vi "NOSAMSNoBouncerDAQrestartFC.vi"(8 "error in (no error)":errorcluster) -> (0 "error out":errorcluster, 2 "Summary Data":T3={"C12LE"=1.472651644671806e-07, "C13LE"=7.43208703350402e-08, "C12"=7.325707563373238e-08, "C13L"=240.0, "C13H"=6.302996266666667, "C1312"=6.305409493333333, "Counts"=0, "LT"=1.0021241544060013, "RT"=0.0, "BadBlocks"=0}, 3 "Run Average Ratios":T7={"C14Rate"=38.07712869341802, "CountErr"=0.06454972243679029, "DT"=0.002413226666666546, "DTfrac"=0.0003827232266545153, "C13"=307109705561.01575, "C13H/L"=0.9856864606602128, "d13C"=-48.24793286826845, "C14/13"=1.23985429323571e-10, "C12Cor"=28715190239906.207, "C13/12"=0.010695028328772694, "C14/12"=1.3260273874313845e-12, "LEC13/12"=0.0} {"LEC13/12" format="%_4e"; "DTfrac" format="%#_3g"; "DT" format="%#_3g"; "CountErr" format="%#_3g"; "d13C" format="%_4g"; "C13/12" format="%_4e"; "C14/12" format="%_4e"; "C14/13" format="%_3e"; "C12Cor" format="%_3e"; "C13" format="%_3e"; "C13H/L" format="%#_3g"})   [LabVIEW 2013]
uses:
  PixieKeithleyDAQstates.ctl
  <vilib>/DAQmx/configure/timing.llb/DAQmx Timing (Sample Clock).vi
  <vilib>/DAQmx/create/channels.llb/DAQmx Create Channel (AI-Voltage-Basic).vi
  <vilib>/DAQmx/create/channels.llb/DAQmx Create Channel (CI-Count Edges).vi
  <vilib>/DAQmx/read.llb/DAQmx Read (Counter U32 1Chan 1Samp).vi
  <resource>/objmgr/daqmx.rc
  <vilib>/DAQmx/configure/trigger.llb/DAQmx Start Trigger (Digital Edge).vi
  <vilib>/DAQmx/read.llb/DAQmx Read (Analog 1D Wfm NChan NSamp).vi
  <vilib>/DAQmx/write.llb/DAQmx Write (Analog Wfm 1Chan NSamp).vi
  <vilib>/DAQmx/create/channels.llb/DAQmx Create Channel (AO-Voltage-Basic).vi
  <vilib>/DAQmx/configure/timing.llb/DAQmx Timing (Use Waveform).vi
  <vilib>/DAQmx/configure/timing.llb/DAQmx Timing (Implicit).vi
  <vilib>/DAQmx/create/channels.llb/DAQmx Create Channel (CO-Pulse Generation-Time).vi
  RunRatios.ctl
  FCOffset.ctl
  SummaryData.ctl
  BouncerParameters.ctl
panel:
  out "Waveform Chart":waveform(dbl)[](graph)
  out "Bouncer Waveform":waveform(dbl)(graph)
  in  "Bouncer Parameters":T1={"12C Period"=1.0, "12C Delay"=0.0, "12C Voltage"=9.022, "13C Period"=10.0, "13C Delay"=0.0, "13C Voltage"=5.239, "14C Period"=100.0, "14C Delay"=0.0, "14C Voltage"=2.0, "LE13C Period"=0.0, "LE13C Delay"=0.0, "LE13C Voltage"=0.0, "LE12C Period"=0.0, "LE12C Delay"=0.0, "LE12C Voltage"=0.0} {"LE12C Voltage" format="%_4f"; "LE13C Voltage" format="%_4f"}
  out "CH1 GDT":dbl
  out "CH0 GDT":dbl
  in  "FC Offset":T2={"HE 12C Offset"=0.0, "HE 13CL Offset"=0.0, "HE 13CH Offset"=0.0, "LE FC Scale"=0, "HE C12 Scale"=0, "HE C13 Scale"=18} {"HE C13 Scale" items=["500 mA/V", "200 mA/V", "100 mA/V", "50 mA/V", "20 mA/V", "10 mA/V", "5 mA/V", "2 mA/V", "1 mA/V", "500 uA/V", "200 uA/V", "100 uA/V", "50 uA/V", "20 uA/V", "10 uA/V", "5 uA/V", "2 uA/V", "1 uA/V", "500 nA/V", "200 nA/V", "100 nA/V", "50 nA/V", "20 nA/V", "10 nA/V", "5 nA/V", "2 nA/V", "1 nA/V", "500 pA/V", "200 pA/V", "100 pA/V", "50 pA/V", "20 pA/V", "10 pA/V", "5 pA/V", "2 pA/V", "1 pA/V", ""]; "HE C12 Scale" items=["500 mA/V", "200 mA/V", "100 mA/V", "50 mA/V", "20 mA/V", "10 mA/V", "5 mA/V", "2 mA/V", "1 mA/V", "500 uA/V", "200 uA/V", "100 uA/V", "50 uA/V", "20 uA/V", "10 uA/V", "5 uA/V", "2 uA/V", "1 uA/V", "500 nA/V", "200 nA/V", "100 nA/V", "50 nA/V", "20 nA/V", "10 nA/V", "5 nA/V", "2 nA/V", "1 nA/V", "500 pA/V", "200 pA/V", "100 pA/V", "50 pA/V", "20 pA/V", "10 pA/V", "5 pA/V", "2 pA/V", "1 pA/V", ""]; "LE FC Scale" items=["500 mA/V", "200 mA/V", "100 mA/V", "50 mA/V", "20 mA/V", "10 mA/V", "5 mA/V", "2 mA/V", "1 mA/V", "500 uA/V", "200 uA/V", "100 uA/V", "50 uA/V", "20 uA/V", "10 uA/V", "5 uA/V", "2 uA/V", "1 uA/V", "500 nA/V", "200 nA/V", "100 nA/V", "50 nA/V", "20 nA/V", "10 nA/V", "5 nA/V", "2 nA/V", "1 nA/V", "500 pA/V", "200 pA/V", "100 pA/V", "50 pA/V", "20 pA/V", "10 pA/V", "5 pA/V", "2 pA/V", "1 pA/V", ""]}
  out "HE 13CL Cup":waveform(dbl)(graph)={"t0"=timestamp(3415120333.4017754 s since 1904-01-01), "dt"=9.999999999999972e-06, "Y"=[0.41889009921070675, 0.6410939957678486, 0.7270772818431984, 0.7261111773784867, 0.7270772818431984, 0.7293315256055366, 0.7267552470213039, 0.7286874559575331, 0.7306196649054364, 0.7254671077369653, 0.7283654211340178, 0.7302976300799747, 0.7277213514879598, 0.7261111773784867, 0.7306196649054364, 0.7341620480069433, 0.7293315256055366, 0.7302976300799747, 0.7319078042105287, 0.7331959435208164, 0.7280433863108267, 0.7331959435208164, 0.7290094907813727, 0.7299755952548376, 0.7309416997312226, 0.7344840828363023, 0.7293315256055366, 0.7299755952548376, 0.7267552470213039, 0.7338400131779094, 0.7219247247317432, 0.7225687943661443, 0.7280433863108267, 0.7280433863108267, 0.7309416997312226, 0.7290094907813727, 0.7328739086927573, 0.7277213514879598, 0.7161280980802982, 0.7286874559575331], "attributes"=variant("NI_ChannelName"=variant(string "PXI1Slot2/ai2"), "NI_UnitDescription"=variant(string "Volts"))}
  out "Bouncer":waveform(dbl)(graph)={"t0"=timestamp(3415120333.4009705 s since 1904-01-01), "dt"=9.999999999999972e-06, "Y"=array[1000 elements], "attributes"=variant("NI_ChannelName"=variant(string "PXI1Slot2/ai0"), "NI_UnitDescription"=variant(string "Volts"))}
  out "LE 13C Cup":waveform(dbl)(graph)={"t0"=timestamp(3415120333.402178 s since 1904-01-01), "dt"=9.999999999999972e-06, "Y"=[0.8050097183722652, 0.24660166407635983, 0.028584441505206795, 0.009584422869030943, 0.009906457076575987, 0.00797425183471986, 0.00797425183471986, 0.007008149216862962, 0.012804764954733521, 0.01312679916455761, 0.010550525492349248, 0.010872559700577551, 0.009584422869030943, 0.01022849128434874, 0.01151662811771772, 0.010872559700577551, 0.010872559700577551, 0.010872559700577551, 0.01022849128434874, 0.009262388661713566, 0.004109841375562904, 0.009262388661713566, 0.01151662811771772, 0.01022849128434874, 0.019567483409006912, 0.01151662811771772, 0.010872559700577551, 0.009906457076575987, 0.009584422869030943, 0.01022849128434874, 0.013448833374609843, 0.01022849128434874, 0.009906457076575987, 0.010550525492349248, 0.00668611501136536, 0.010550525492349248, 0.01022849128434874, 0.01022849128434874, 0.009584422869030943, 0.013448833374609843], "attributes"=variant("NI_ChannelName"=variant(string "PXI1Slot2/ai3"), "NI_UnitDescription"=variant(string "Volts"))}
  out "LE 12C Cup":waveform(dbl)(graph)={"t0"=timestamp(3415120333.4013777 s since 1904-01-01), "dt"=9.999999999999972e-06, "Y"=[0.00668611501136536, 0.007008149216862962, 0.007652217628540168, 0.007330183422587883, 0.00861832024776164, 0.007330183422587883, 0.009262388661713566, 0.01312679916455761, 0.05338107720327494, 0.6781279926088322, 0.8175690797952145, 0.8223996035554544, 0.8240097781590372, 0.8233657083165931, 0.8249758829252316, 0.8230436733958766, 0.8243318130807649, 0.8236877432376466, 0.8243318130807649, 0.8243318130807649, 0.8233657083165931, 0.8278741972420289, 0.8236877432376466, 0.8240097781590372, 0.8227216384754971, 0.8246538480028296, 0.8246538480028296, 0.8246538480028296, 0.8249758829252316, 0.8252979178479707, 0.8214334987973474, 0.8236877432376466, 0.8246538480028296, 0.8246538480028296, 0.8227216384754971, 0.8236877432376466, 0.8243318130807649, 0.8217555337163797, 0.8240097781590372, 0.8243318130807649], "attributes"=variant("NI_ChannelName"=variant(string "PXI1Slot2/ai3"), "NI_UnitDescription"=variant(string "Volts"))}
  out "HE 13CH Cup":waveform(dbl)(graph)={"t0"=timestamp(3415120333.4017754 s since 1904-01-01), "dt"=9.999999999999972e-06, "Y"=[0.41889009921070675, 0.6410939957678486, 0.7270772818431984, 0.7261111773784867, 0.7270772818431984, 0.7293315256055366, 0.7267552470213039, 0.7286874559575331, 0.7306196649054364, 0.7254671077369653, 0.7283654211340178, 0.7302976300799747, 0.7277213514879598, 0.7261111773784867, 0.7306196649054364, 0.7341620480069433, 0.7293315256055366, 0.7302976300799747, 0.7319078042105287, 0.7331959435208164, 0.7280433863108267, 0.7331959435208164, 0.7290094907813727, 0.7299755952548376, 0.7309416997312226, 0.7344840828363023, 0.7293315256055366, 0.7299755952548376, 0.7267552470213039, 0.7338400131779094, 0.7219247247317432, 0.7225687943661443, 0.7280433863108267, 0.7280433863108267, 0.7309416997312226, 0.7290094907813727, 0.7328739086927573, 0.7277213514879598, 0.7161280980802982, 0.7286874559575331], "attributes"=variant("NI_ChannelName"=variant(string "PXI1Slot2/ai2"), "NI_UnitDescription"=variant(string "Volts"))}
  out "HE 12C Cup":waveform(dbl)(graph)={"t0"=timestamp(3415120333.400973 s since 1904-01-01), "dt"=9.999999999999972e-06, "Y"=[-0.00168677425192447, 0.003143738765882537, -0.002652876849375083, -0.00168677425192447, 0.0008894993512310448, -0.002652876849375083, 0.0005674651500443148, -0.000720671652438485, 0.0018556019561503992, 0.0018556019561503992, 0.0024996703605630385, 0.0015335677542840436, 0.002177636158243383, -0.0013647400523220184, 0.005397978191647298, 0.0018556019561503992, 0.0012115335526442733, 0.0015335677542840436, 0.016669175487689536, 0.2607711773435167, 0.6375516136789285, 0.6369075442122739, 0.6423821347186465, 0.6456024821175347, 0.6449584126352536, 0.6423821347186465, 0.6456024821175347, 0.6427041694571275, 0.639805856822051, 0.6427041694571275, 0.6388397526159826, 0.6449584126352536, 0.6423821347186465, 0.6443143431542244, 0.6452804473762376, 0.6401278915580318, 0.6410939957678486, 0.6468906210858548, 0.6446363778945825, 0.6433482389350278], "attributes"=variant("NI_ChannelName"=variant(string "PXI1Slot2/ai1"), "NI_UnitDescription"=variant(string "Volts"))}
  out "C13LE":dbl=7.360825676338929e-08 format="%_4g"
  out "C12LE":dbl=7.360825676338929e-08 format="%_4g"
  in  "SampClk.Rate":dbl=10000.0
  out "DT Corrected Rate":dbl=38.103932081925684
  out "SCA Rate":dbl=38.473667612740456
  out "SCA Counts":u32=244
  out "CH1 SFDT":dbl=0.004433706666666666 format="%#_2f"
  out "CH0 SFDT":dbl=0.004324053333333333 format="%#_2f"
  in  "Mode":enum16{"Tuning", "Run", "Manual"}(ring)
  out "Block Spectrum":u32[][](graph) caption="ADC Spectrum"
  out "RunningAverages":T3={"C12LE"=1.4726514132603862e-07, "C13LE"=7.431122697335651e-08, "C12"=7.326197420828519e-08, "C13L"=222.0, "C13H"=5.887767893333334, "C1312"=5.884231466666667, "Counts"=0, "LT"=1.0020921000294485, "RT"=0.0, "BadBlocks"=0}
  out "Elapsed Time":dbl=6.3420000000000005
  out "element":T4=enum."Idle"
  in  "Stop":bool
  in  "Stop DAQ":bool
  in  "Run Parameters":T5={"Block time (s)"=0.2, "Max Runtime (s)"=100000.0, "Max Counts"=100000, "C12 Limit"=-1.0, "Max BadBlocks"=100} {"Block time (s)" min=0.0 max=100.0 step=0.1}
  out "Acquiring":bool
  in  "StartDAQ":bool
  in  "Logfile":string="Feb12.txt"
  in  "Log File Path":path=path "C:/DAQ Logs"
  out "Good Block":bool=TRUE
  out "Currents & Counts":cluster{dbl, dbl, dbl, dbl, dbl}(graph)
  out "Ratios":T6(graph)={"C14/12"=1.3260273874313845e-12, "C14/12"=1.3130784198635677e-12, "d13C"=-48.24793286826845, "d13C"=-48.27837602145524}
  out "13C H/L":dbl(knob)=0.9886607752123965 scale=0.0..2.0 scale format="%#_3g"
  out "Currents":cluster{dbl, dbl}(knob)={1.4754487124301994e-07, 1.4806074705013686e-07} scale=0.0..1e-06 scale format="%#_1e"
  out "12/13":dbl=93.50437948492602
  out "Ch1 Rate 2":cluster{dbl, "Ch1 Rate":dbl}(graph)={38.07712869341802, "Ch1 Rate"=37.7052907013146}
  out "Moving Averages":T7={"C14Rate"=37.7052907013146, "CountErr"=0.06711560552140243, "DT"=-0.0035364266666668698, "DTfrac"=-0.0006010006041910865, "C13"=307099831658.9964, "C13H/L"=0.9858802928197172, "d13C"=-48.27837602145524, "C14/13"=1.2277861077821284e-10, "C12Cor"=28715185727621.875, "C13/12"=0.010694686232971703, "C14/12"=1.3130784198635677e-12, "LEC13/12"=0.0} {"LEC13/12" format="%_4e"; "DTfrac" format="%#_3g"; "DT" format="%#_3g"; "CountErr" format="%#_3g"; "d13C" format="%_4g"; "C13/12" format="%_4e"; "C14/12" format="%_4e"; "C14/13" format="%_3e"; "C12Cor" format="%_3e"; "C13" format="%_3e"; "C13H/L" format="%#_3g"}
  in  "CountPoints":i32=30 min=1
  in  "CurPoints":i32=30 min=1
  out "C12":dbl=1.4754487124301994e-07 format="%_4g"
  out "C13L":dbl=7.445249028674759e-08 format="%_4g"
  out "C13H":dbl=7.360825676338929e-08 format="%_4g"
  out "Run time [s]":dbl=6.305409493333333 format="%_6g"
  out "Ch1 LT":dbl=6.302996266666667
  out "Ch1 Counts":u32=240
  out "Ch1 Rate":dbl=38.07712869341802
  out "Ch0 LT":dbl=6.305354879999999
  out "Ch0 Counts":u32=243
  out "Ch0 Rate":dbl=38.53867143477895
  # "Currents"
  # "Counts"
  # "Livetime"
  # "Rate"
  # "SFDT"
  # "GDT"
  # "Cor Rate"
  # "Ch 0"
  # "Ch1"
  # "SCA"
  # "ms"
  # "us"
  # "kV"
  # "ms"
  # "us"
  # "kV"
  # "ms"
  # "us"
  # "kV"
  # "ms"
  # "us"
  # "kV"
  # "ms"
  # "us"
  # "kV"
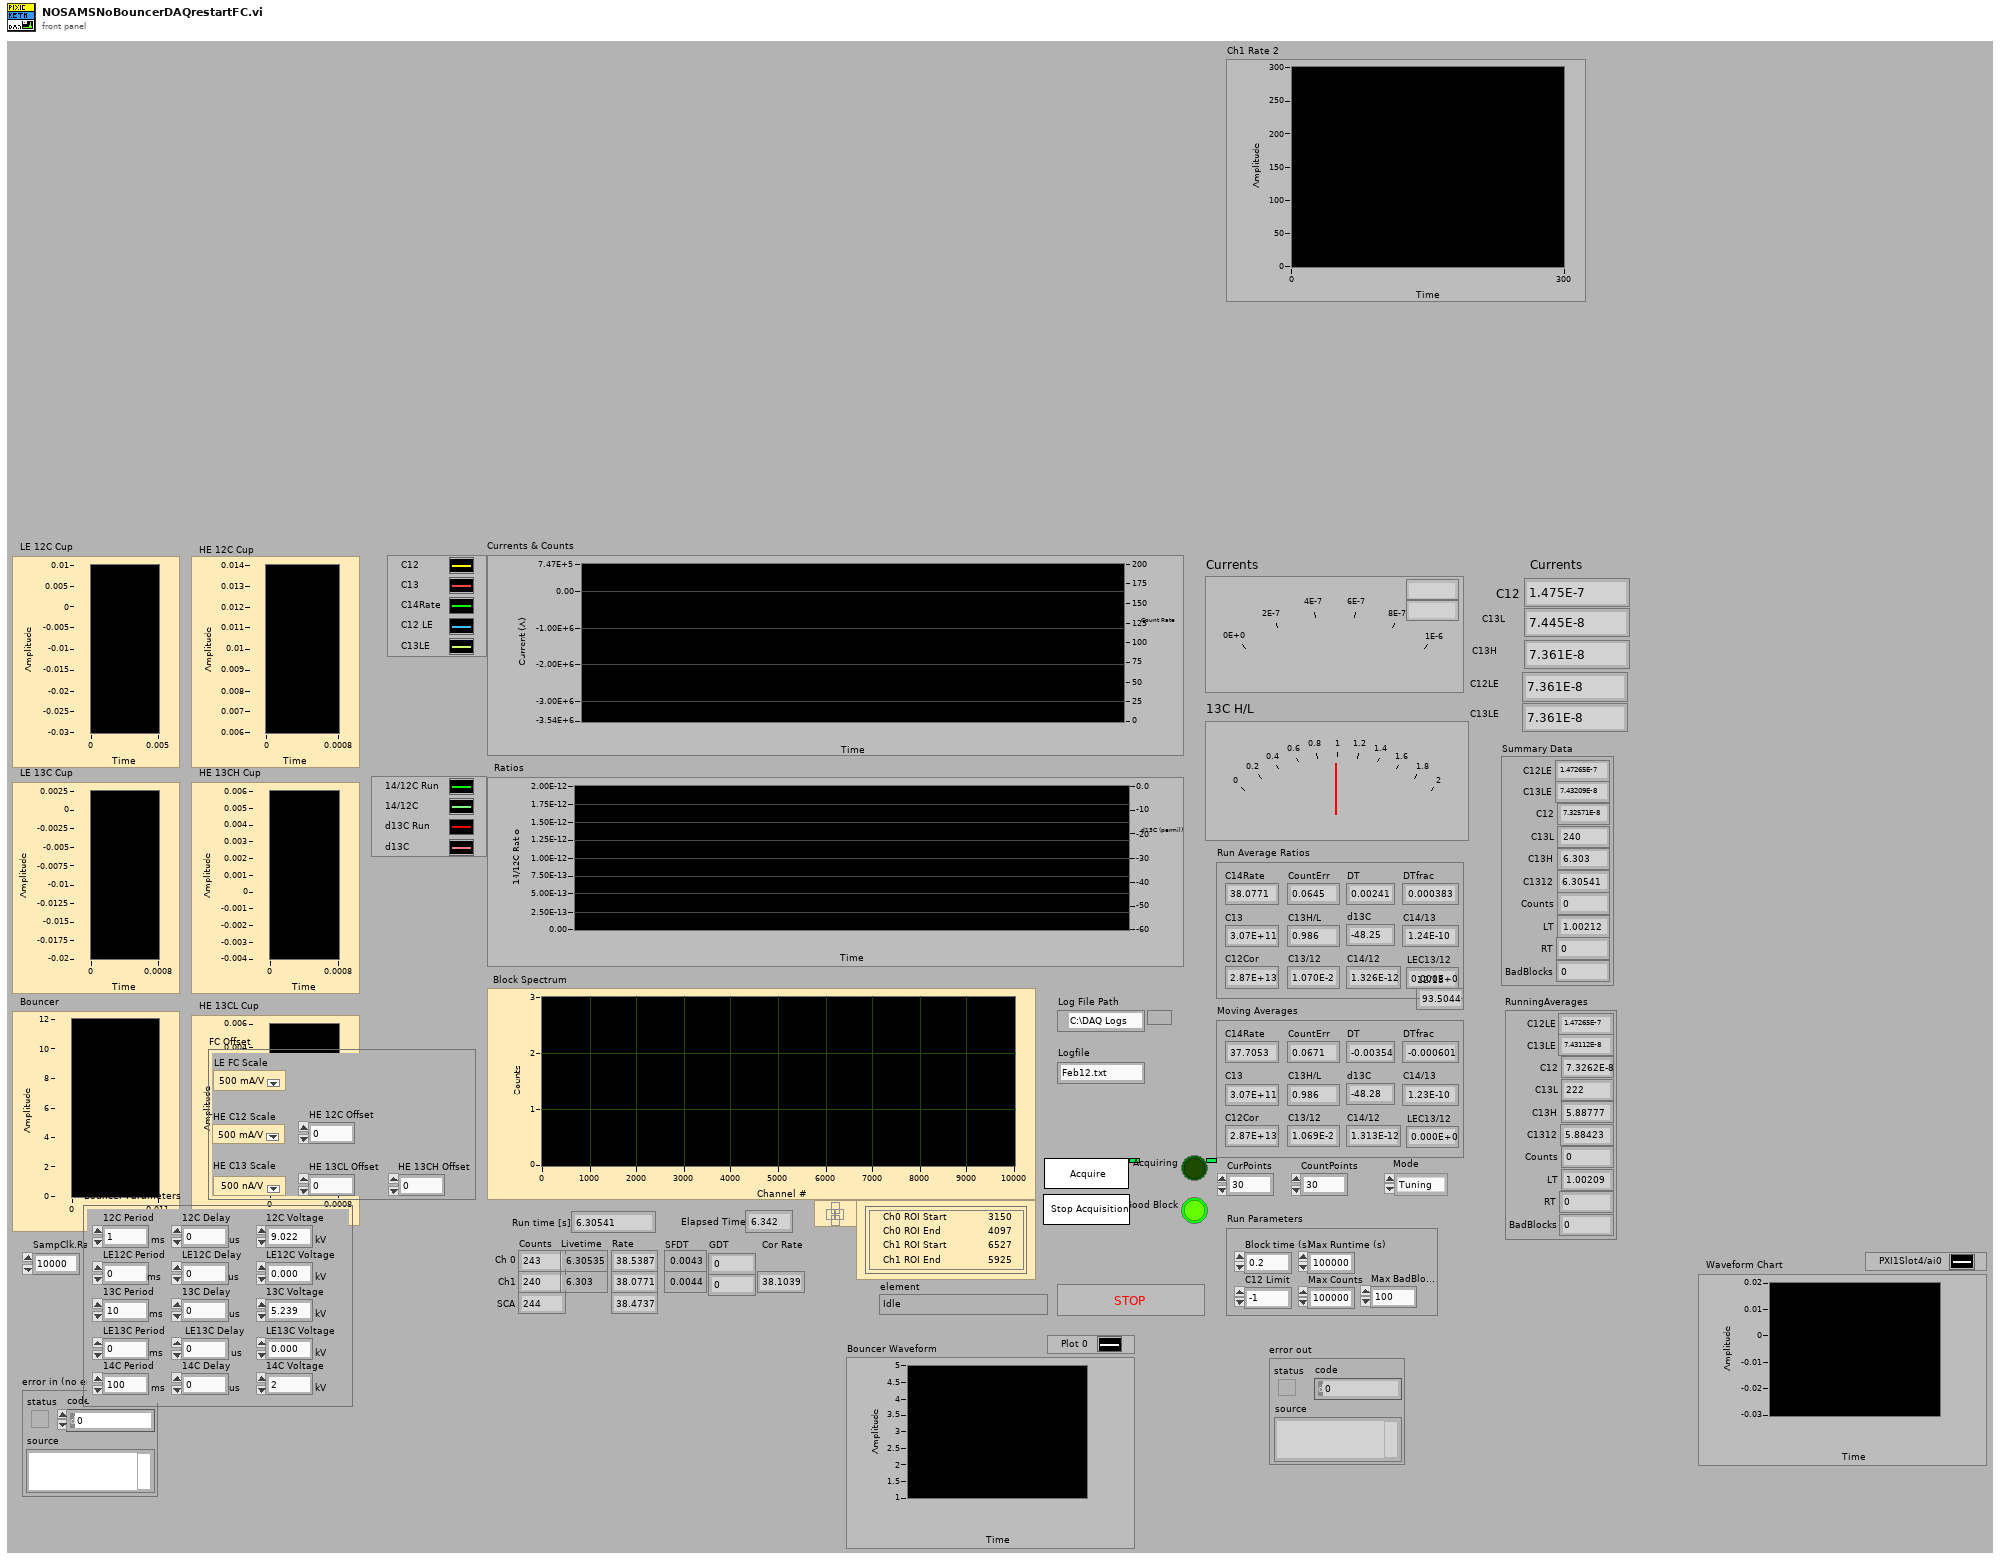
[diagram p1: front panel]
types:
  T1 = typedef "BouncerParameters.ctl" = cluster{"12C Period":dbl, "12C Delay":dbl, "12C Voltage":dbl, "13C Period":dbl, "13C Delay":dbl, "13C Voltage":dbl, "14C Period":dbl, "14C Delay":dbl, "14C Voltage":dbl, "LE13C Period":dbl, "LE13C Delay":dbl, "LE13C Voltage":dbl, "LE12C Period":dbl, "LE12C Delay":dbl, "LE12C Voltage":dbl}
  T2 = typedef "FCOffset.ctl" = cluster{"HE 12C Offset":dbl, "HE 13CL Offset":dbl, "HE 13CH Offset":dbl, "LE FC Scale":u16, "HE C12 Scale":u16, "HE C13 Scale":u16}
  T3 = typedef "SummaryData.ctl" = cluster{"C12LE":dbl, "C13LE":dbl, "C12":dbl, "C13L":dbl, "C13H":dbl, "C1312":dbl, "Counts":u32, "LT":dbl, "RT":dbl, "BadBlocks":u8}
  T4 = typedef "PixieKeithleyDAQstates.ctl" = enum16{"Initialize", "Restart Bouncer", "Idle", "Load Wheel", "Load Sample", "Start Run", "Wait", "Get Block", "Check Data", "Check Run", "Check Sample", "Analyse and Display", "Stop DAQ", "Log Data", "Stop"}
  T5 = cluster{"Block time (s)":dbl, "Max Runtime (s)":dbl, "Max Counts":u32, "C12 Limit":dbl, "Max BadBlocks":u8}
  T6 = cluster{"C14/12":dbl, "C14/12":dbl, "d13C":dbl, "d13C":dbl}
  T7 = typedef "RunRatios.ctl" = cluster{"C14Rate":dbl, "CountErr":dbl, "DT":dbl, "DTfrac":dbl, "C13":dbl, "C13H/L":dbl, "d13C":dbl, "C14/13":dbl, "C12Cor":dbl, "C13/12":dbl, "C14/12":dbl, "LEC13/12":dbl}
  T8 = typedef "BlockData.ctl" = cluster{"LE C12":dbl[], "LE C13":dbl[], "C12":dbl[], "C13L":dbl[], "C13H":dbl[], "C1312":dbl[], "Counts":u32[], "LT":dbl[], "RT":dbl[]}
  T9 = typedef "PixieTimes.ctl" = cluster{"CH0 LT":dbl, "CH1 LT":dbl, "CH0 SFDT":dbl, "CH1 SFDT":dbl, "CH0 GDT":dbl, "CH1 GDT":dbl, "Run time [s]":dbl}
  T10 = typedef "LVCursorListTypeDef.ctl" = cluster{"Name":string, "Color":u32, "Style":u8, "Point Style":u8, "Name Visible":bool, "Allow Drag":bool, "Cursor Mode":u32, "Plot":i32, "Index":i32, "Position":cluster{"X":dbl, "Y":dbl}, "X Scale":u32, "Y Scale":u32, "Watch Plots":i32[], "Watch All Plots":bool, "Plot Area":i32, "Label Offset":cluster{"X":dbl, "Y":dbl}}[]
  T11 = cluster{"Ch0 Counts":u32, "Ch0 Rate":dbl, "Ch1 Counts":u32, "Ch1 Rate":dbl}
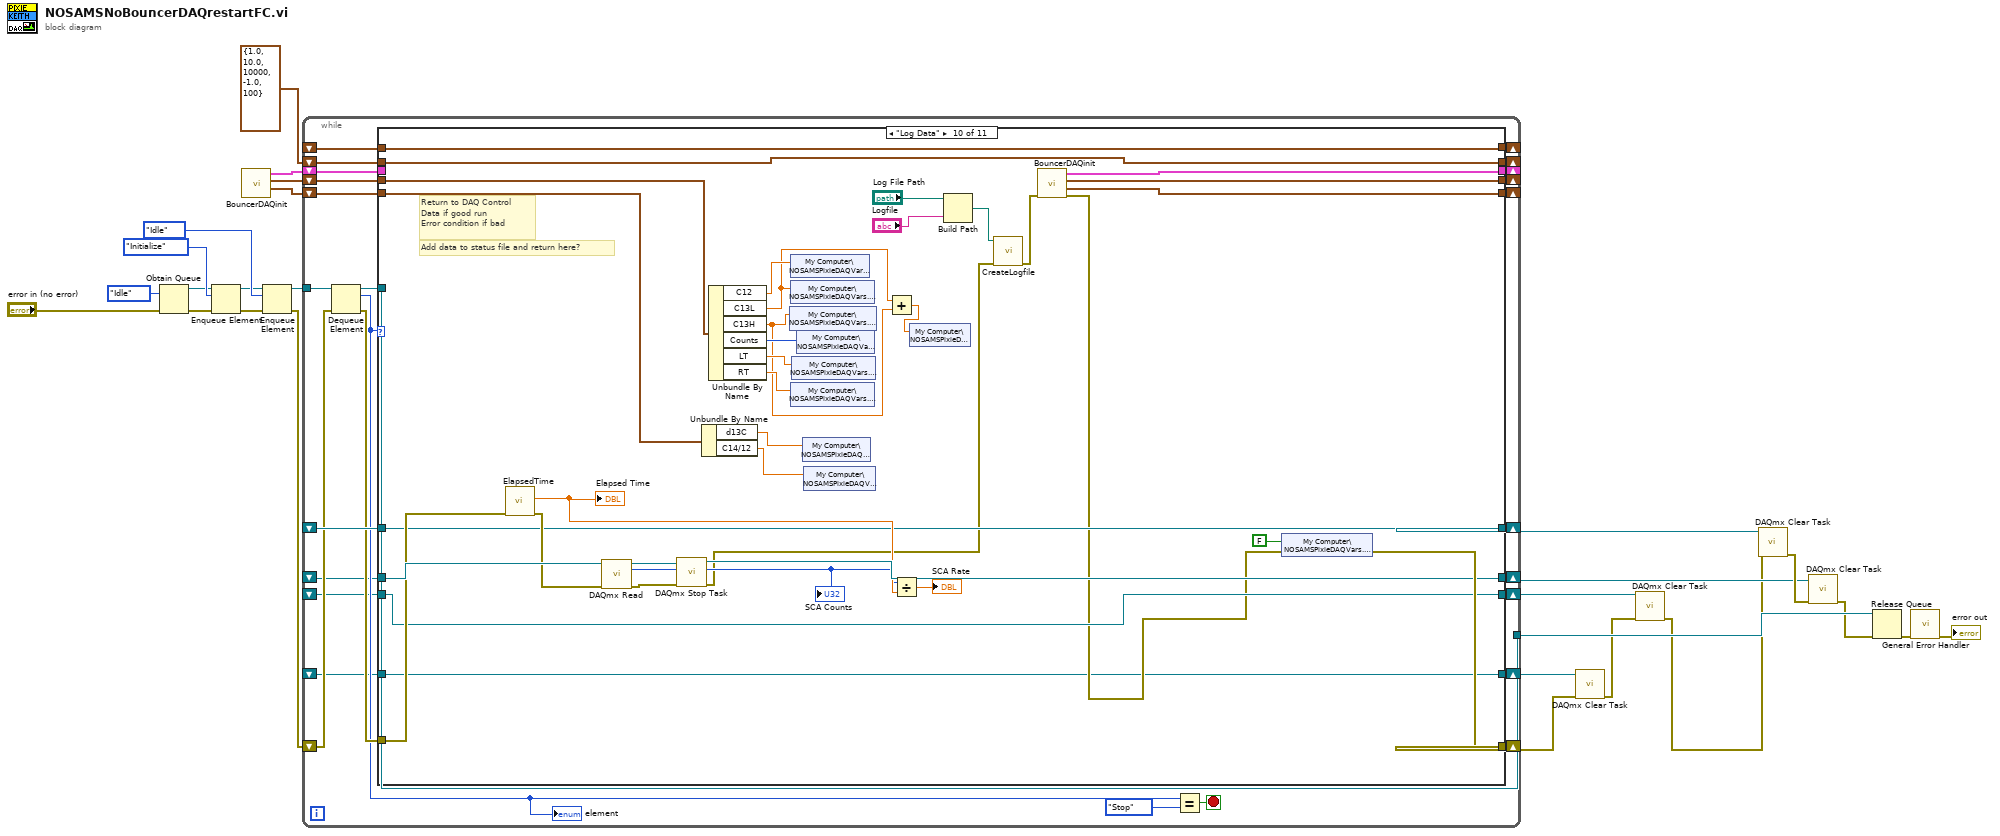
[diagram p0: block diagram]
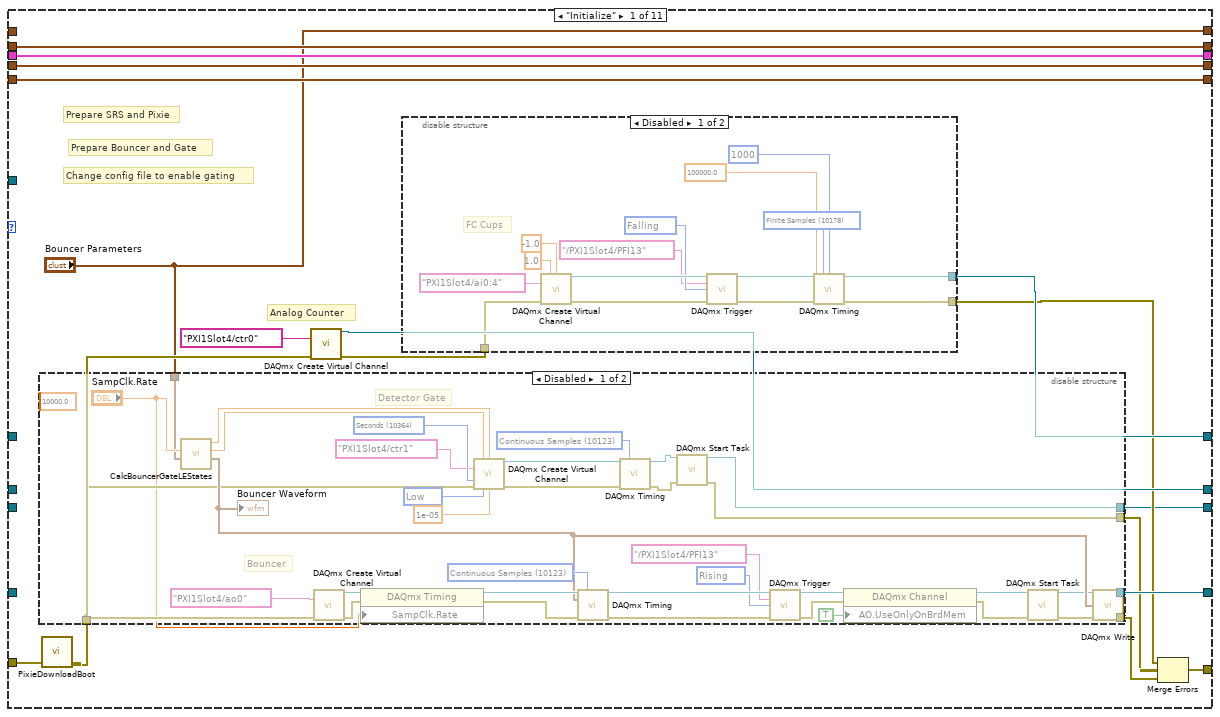
[diagram p2: hidden frame]
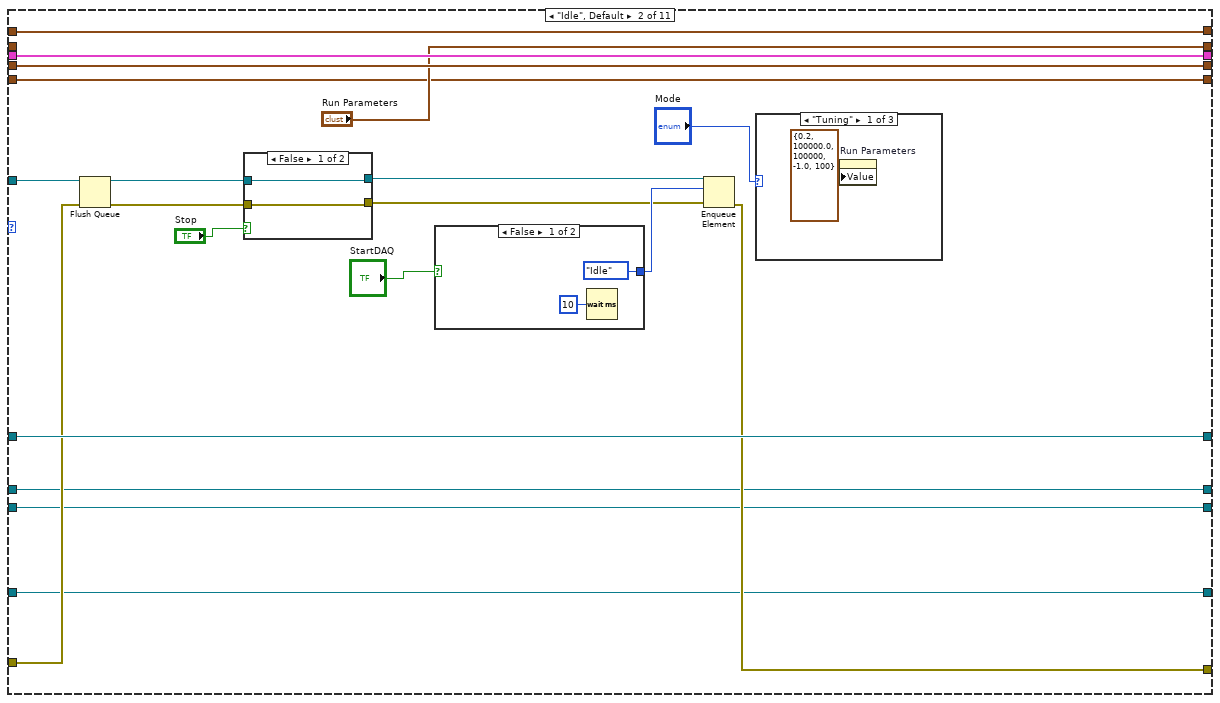
[diagram p5: hidden frame]
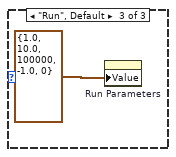
[diagram p7: hidden frame]
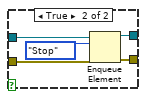
[diagram p8: hidden frame]
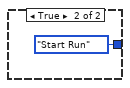
[diagram p9: hidden frame]
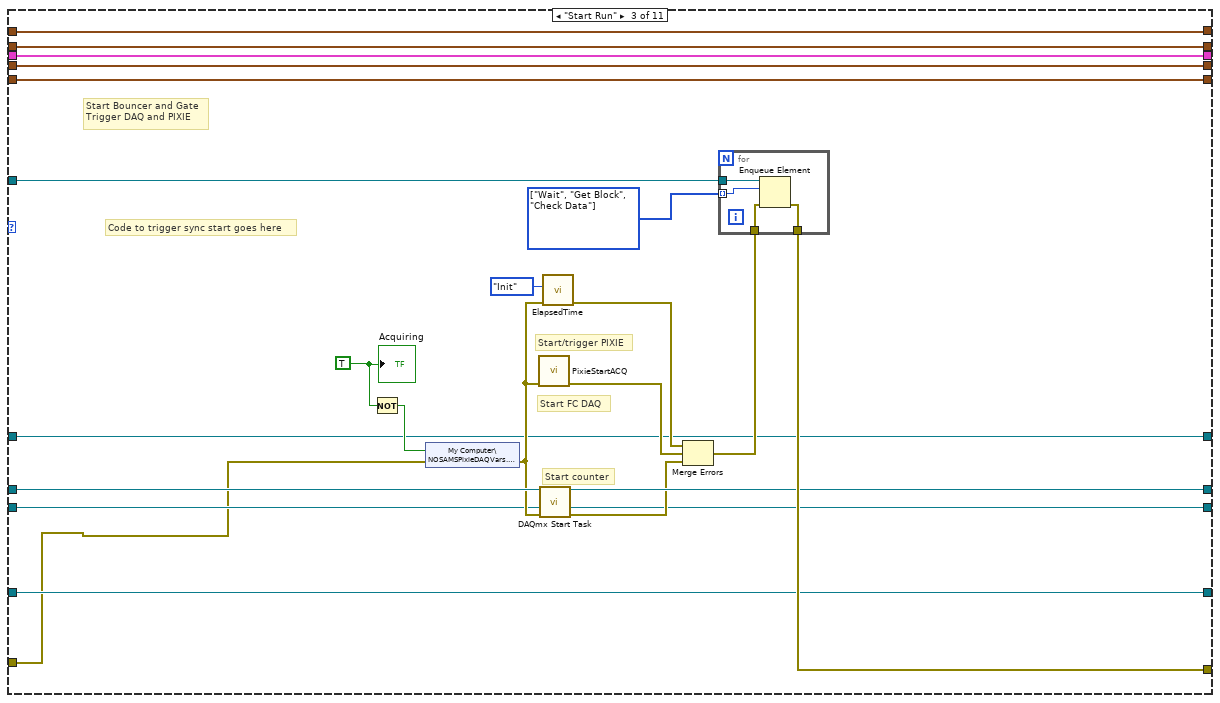
[diagram p10: hidden frame]
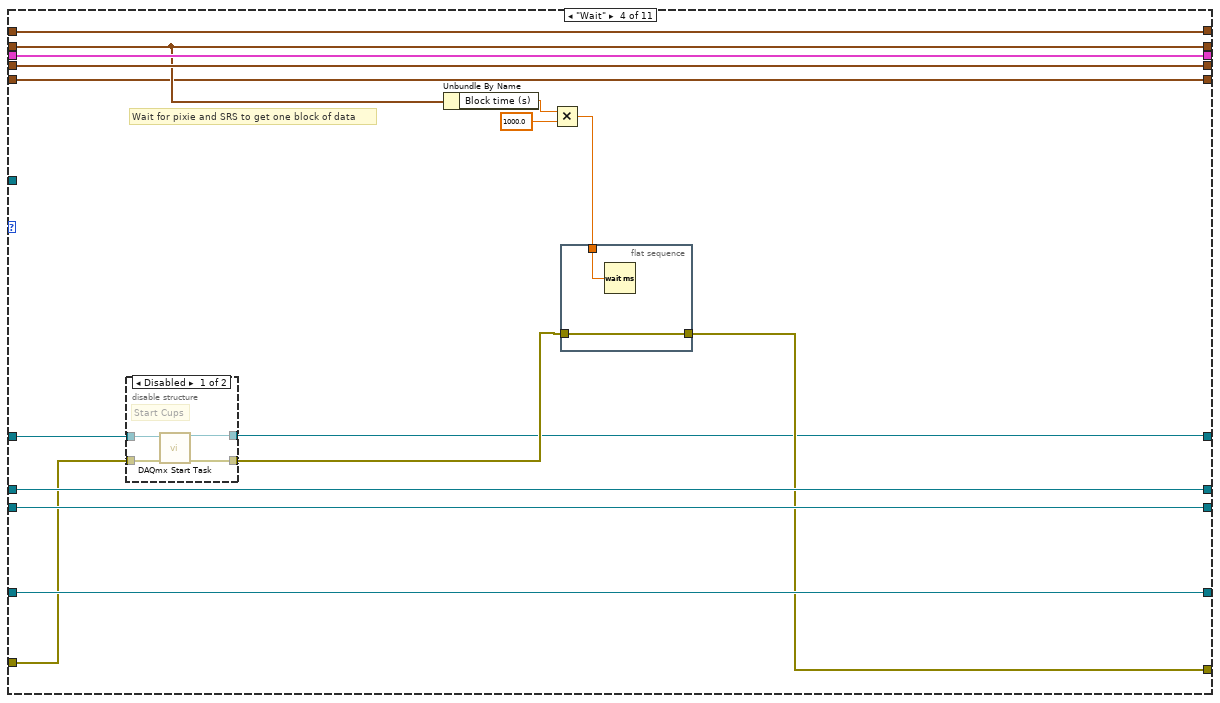
[diagram p11: hidden frame]
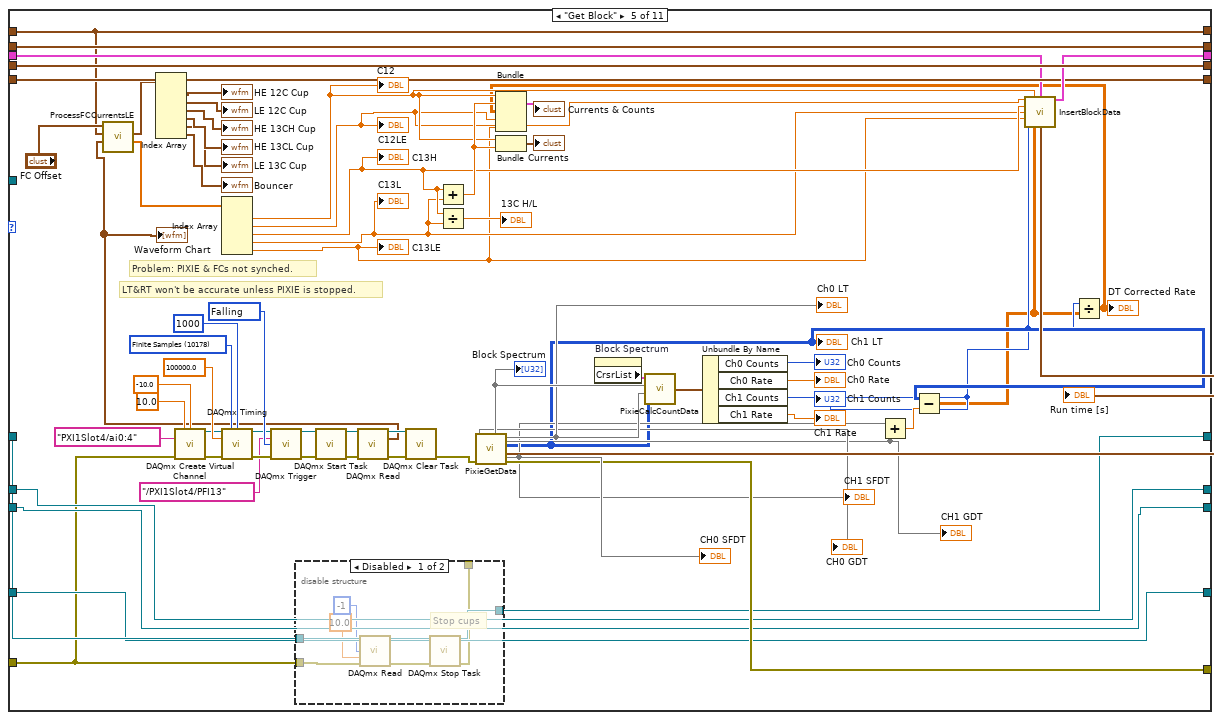
[diagram p13: hidden frame]
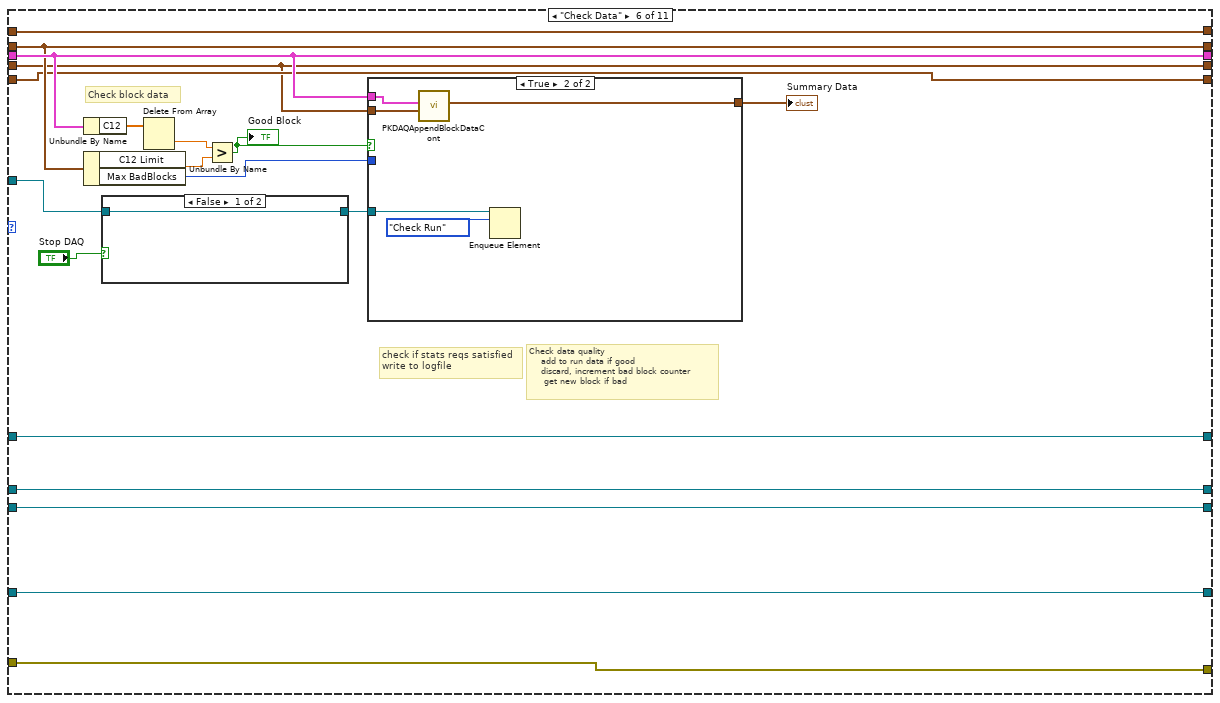
[diagram p15: hidden frame]
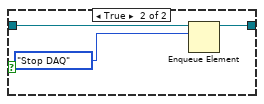
[diagram p16: hidden frame]
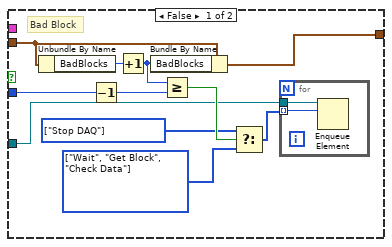
[diagram p17: hidden frame]
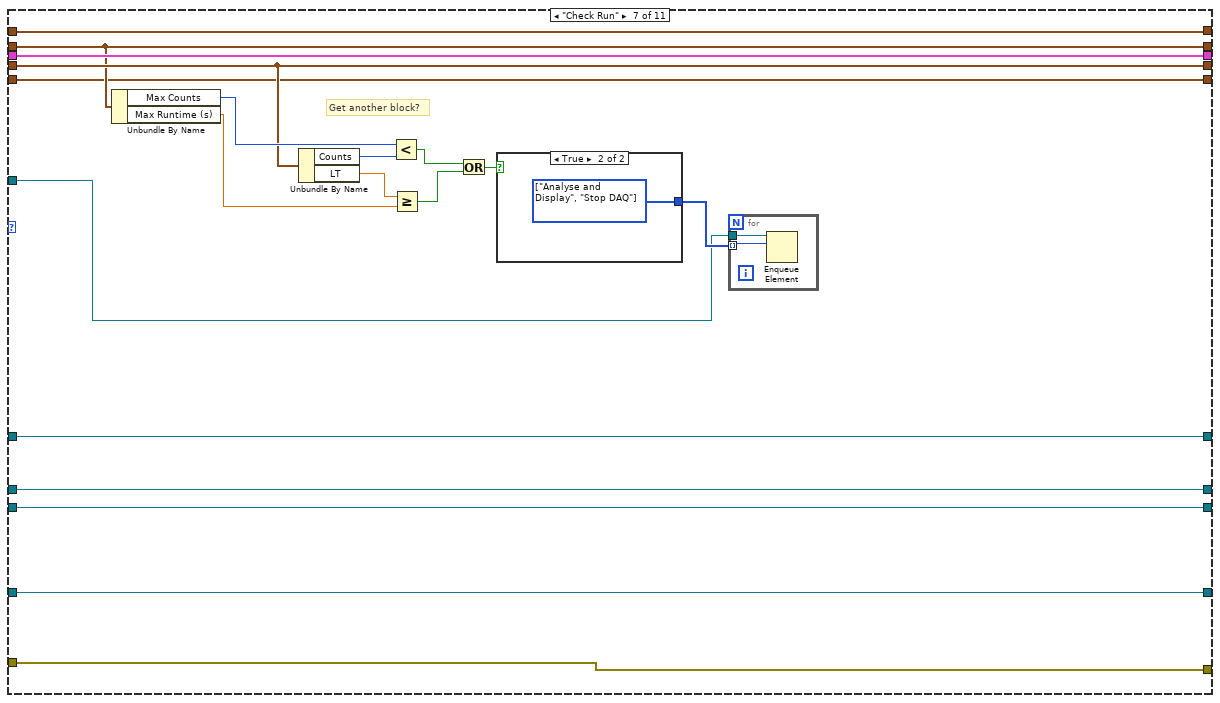
[diagram p18: hidden frame]
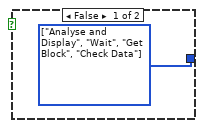
[diagram p19: hidden frame]
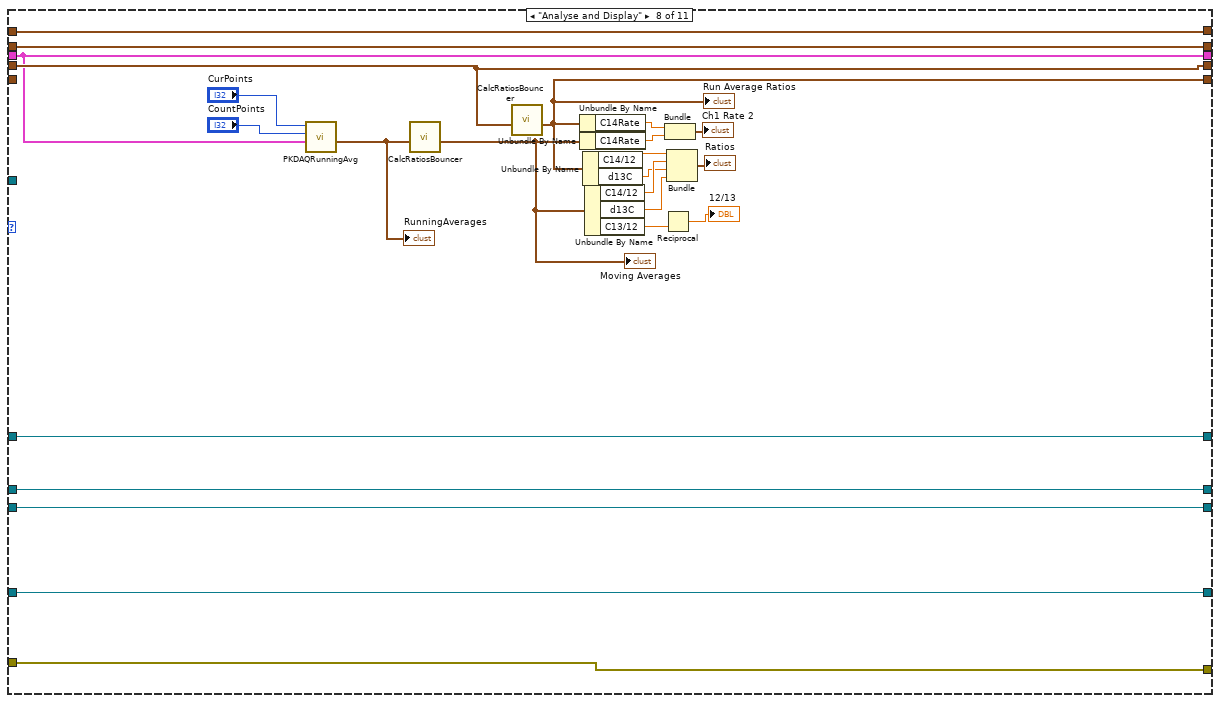
[diagram p20: hidden frame]
diagram:
  n1 = Obtain Queue(element data type=PixieKeithleyDAQstates."Idle" ("Next State"), error in (no error)="error in (no error)") -> (queue out=w16:refnum<queue>, error out=w15:errorcluster)  [unwired: 2 in, 2 out]
  n2 = Enqueue Element(queue=w16, element=PixieKeithleyDAQstates."Initialize", error in (no error)=w15) -> (queue out=w18:refnum<queue>, error out=w17:errorcluster)  [unwired: 2 out]
  n3 = call "BouncerDAQinit.vi"() -> ("Run Ratios"=w11:T7, "Summary Data"=w10:T3, "Block Data"=w9:T8)  [unwired: 2 in, 7 out]
  n4 = Enqueue Element(queue=w18, element=PixieKeithleyDAQstates."Idle", error in (no error)=w17) -> (queue out=w23:refnum<queue>, error out=w22:errorcluster)  [unwired: 2 out]
  n5 = while {
    shift-right: [w48] -> _
    shift-left: w9 -> [w49]
    shift-right: [w46] -> _
    shift-left: w10 -> [w47]
    shift-right: [w45] -> w26
    shift-left: _ -> [w44]
    shift-right: [w50] -> w2
    shift-left: w22 -> [w41]
    tunnel: w23 -> [w43]
    tunnel: [w40] -> w20
    shift-right: [w39] -> _
    shift-left: T5 {"Block time (s)"=1.0, "Max Runtime (s)"=10.0, "Max Counts"=10000, "C12 Limit"=-1.0, "Max BadBlocks"=100} ("Run Parameters 2") -> [w38]
    shift-right: [w35] -> _
    shift-left: w11 -> [w36]
    shift-right: [w34] -> w6
    shift-left: _ -> [w33]
    shift-right: [w32] -> w4
    shift-left: _ -> [w29]
    shift-right: [w31] -> w5
    shift-left: _ -> [w30]
    shift-right: [w28] -> _
    shift-left: _ -> [w27]
    stop <- w52 stop-if-true
    n6 = Dequeue Element(queue=w43, error in (no error)=w41) -> (queue out=w40:refnum<queue>, element=w37:T4, error out=w42:errorcluster)  [unwired: 2 out]
    "element" <- w37
    n7 = case shown="\"Log Data\"" w37 {
      tunnel: [w59 w132 w165 w182 w246 w295 w336 w364 w370 w413 w427] -> w50
      tunnel: w42 -> [w67 w134 w154 w183 w203 w295 w336 w364 w372 w396 w427]
      tunnel: w49 -> [w69 w140 w174 w194 w247 w289 w332 w342 w378 _ w432]
      tunnel: [w69 w140 w174 w194 w264 w289 w332 w342 w378 w407 w432] -> w48
      tunnel: w47 -> [w68 w139 w173 w193 w265 w278 w329 w343 w377 w391 w431]
      tunnel: [w68 w139 w173 w193 w265 w278 w329 w343 w377 w408 w431] -> w46
      tunnel: w38 -> [w66 _ w164 w189 w258 w285 w325 w348 w371 w415 w426]
      tunnel: [w57 w138 w157 w180 w223 w293 w333 w363 w373 w390 w428] -> w45
      tunnel: w44 -> [_ w138 w157 w181 w268 w293 w333 w363 w373 w390 w428]
      tunnel: w40 -> [_ w137 w169 _ _ w287 w323 _ w374 _ w429]
      tunnel: [w66 "Run Parameters" w164 w189 w258 w285 w325 w348 w371 w415 w426] -> w39
      tunnel: w36 -> [w65 w125 w162 w188 w256 w283 w322 _ w369 w406 w425]
      tunnel: [w65 w125 w162 w188 w256 w283 w322 w347 w369 w409 w425] -> w35
      tunnel: [w63 w124 w160 w187 w245 w282 w321 w346 w368 w397 w424] -> w34
      tunnel: w33 -> [_ w124 w161 w187 w245 w282 w321 w346 w368 w400 w424]
      tunnel: [w61 w122 w156 w185 w243 w280 w319 w344 w366 w386 w422] -> w32
      tunnel: [w55 w123 w155 w186 w244 w281 w320 w345 w367 w388 w423] -> w31
      tunnel: w30 -> [_ w123 w155 w186 w244 w281 w320 w345 w367 w388 w423]
      tunnel: w29 -> [_ w122 w156 w185 w243 w280 w319 w344 w366 w386 w422]
      tunnel: ["Bouncer Parameters" w121 w153 w179 w222 w277 w318 w341 w365 w385 w421] -> w28
      tunnel: w27 -> [_ w121 w153 w179 w222 w277 w318 w341 w365 w385 w421]
      frame "Initialize" {
        # "Analog Counter"
        # "Change config file to enable gating"
        # "Prepare Bouncer and Gate"
        # "Prepare SRS and Pixie"
        n8 = call "PixieDownloadBoot.vi"("error in (no error)"=w67) -> ("error out"=w58:errorcluster)  [unwired: 5 in, 5 out]
        n9 = disable-structure shown="Disabled" {
          disable-tunnel: [w98 _] -> w61
          disable-tunnel: [w96 _] -> w60
          disable-tunnel: w58 -> [w95 _]
          disable-tunnel: [w88 _] -> w55
          disable-tunnel: [w86 _] -> w54
          disable-tunnel: "Bouncer Parameters" -> [w85 _]
          frame Disabled {
            w108 = 10280 items=["Rising"=10280, "Falling"=10171] ("edge")
            w111 = 10123 items=["Finite Samples"=10178, "Continuous Samples"=10123] ("sample mode")
            w114 = 10123 items=["Finite Samples"=10178, "Continuous Samples"=10123, "Hardware Timed Single Point"=12522] ("sample mode")
            w119 = 10214 items=["High"=10192, "Low"=10214] ("idle state")
            w118 = 10364 items=["Seconds"=10364] ("units")
            (unwired) 10000.0 ("rate")
            # "Bouncer"
            # "Detector Gate"
            n10 = call "CalcBouncerGateLEStates.vi"("Bouncer Settings"=w85, "SampClk.Rate"="SampClk.Rate") -> ("Bouncer Waveform"=w97:waveform(dbl), "High time"=w112:dbl, "low time"=w113:dbl)  [unwired: 7 in]
            "Bouncer Waveform" <- w97
            n11 = call-poly <vilib>:"DAQmx Create Virtual Channel.vi"("physical channels"=tag "PXI1Slot4/ao0", "error in"=w95) -> ("task out"=w102:refnum<k21>, "error out"=w103:errorcluster)  [unwired: 7 in, 5 out]
            n12 = property class="DAQmx Timing"(reference=w102, error in=w103, "SampClk.Rate"="SampClk.Rate") -> (reference out=w101:refnum<k21>, error out=w100:errorcluster)
            n13 = call-poly <vilib>:"DAQmx Create Virtual Channel.vi"("high time"=w112, "low time"=w113, "counter"=tag "PXI1Slot4/ctr1", "units"=w118, "error in"=w95, "idle state"=w119, "initial delay"=1e-05) -> ("task out"=w115:refnum<k21>, "error out"=w116:errorcluster)  [unwired: 2 in, 5 out]
            n14 = call-poly <vilib>:"DAQmx Timing.vi"("task/channels in"=w101, "sample mode"=w111, "waveform"=w97, "error in"=w100) -> ("task out"=w110:refnum<k21>, "error out"=w109:errorcluster)  [unwired: 10 out]
            n15 = call-poly <vilib>:"DAQmx Timing.vi"("task/channels in"=w115, "sample mode"=w114, "error in"=w116) -> ("task out"=w89:refnum<k21>, "error out"=w87:errorcluster)  [unwired: 1 in, 10 out]
            n16 = call <vilib>:"DAQmx Start Task.vi"("task/channels in"=w89, "error in"=w87) -> ("task out"=w88:refnum<k21>, "error out"=w86:errorcluster)  [unwired: 12 in]
            n17 = call-poly <vilib>:"DAQmx Trigger.vi"("task/channels in"=w110, "source"=tag "/PXI1Slot4/PFI13", "edge"=w108, "error in"=w109) -> ("task out"=w105:refnum<k21>, "error out"=w104:errorcluster)  [unwired: 10 out]
            n18 = property class="DAQmx Channel"(reference=w105, error in=w104, "AO.UseOnlyOnBrdMem"=TRUE) -> (reference out=w93:refnum<k21>, error out=w91:errorcluster)
            n19 = call <vilib>:"DAQmx Start Task.vi"("task/channels in"=w93, "error in"=w91) -> ("task out"=w92:refnum<k21>, "error out"=w90:errorcluster)  [unwired: 12 in]
            n20 = call-poly <vilib>:"DAQmx Write.vi"("task/channels in"=w92, "data"=w97, "error in"=w90) -> ("task out"=w98:refnum<k21>, "error out"=w96:errorcluster)  [unwired: 1 in, 10 out]
          }
          frame Enabled {
          }
        }
        n21 = call-poly <vilib>:"DAQmx Create Virtual Channel.vi"("counter"=tag "PXI1Slot4/ctr0" ("Counter(s)"), "error in"=w58) -> ("task out"=w63:refnum<k21>, "error out"=w62:errorcluster)  [unwired: 5 in, 7 out]
        n22 = disable-structure shown="Disabled" {
          disable-tunnel: w62 -> [w80 _]
          disable-tunnel: [w73 _] -> w57
          disable-tunnel: [w72 _] -> w56
          frame Disabled {
            w75 = 10171 items=["Rising"=10280, "Falling"=10171] ("edge")
            w81 = 10178 items=["Finite Samples"=10178, "Continuous Samples"=10123] ("sample mode")
            # "FC Cups"
            n23 = call-poly <vilib>:"DAQmx Create Virtual Channel.vi"("maximum value"=1.0, "minimum value"=-1.0, "physical channels"=tag "PXI1Slot4/ai0:4", "error in"=w80) -> ("task out"=w79:refnum<k21>, "error out"=w77:errorcluster)  [unwired: 5 in, 5 out]
            n24 = call-poly <vilib>:"DAQmx Trigger.vi"("task/channels in"=w79, "source"=tag "/PXI1Slot4/PFI13", "edge"=w75, "error in"=w77) -> ("task out"=w78:refnum<k21>, "error out"=w76:errorcluster)  [unwired: 10 in]
            n25 = call-poly <vilib>:"DAQmx Timing.vi"("task/channels in"=w78, "sample mode"=w81, "samples per channel"=1000, "rate"=100000.0, "error in"=w76) -> ("task out"=w73:refnum<k21>, "error out"=w72:errorcluster)  [unwired: 2 in, 7 out]
          }
          frame Enabled {
          }
        }
        n26 = Merge Errors(w56, w54, w60) -> (w59:errorcluster)
      }
      frame "Idle", Default {
        n27 = Flush Queue(queue=w137, error in (no error)=w134) -> (queue out=w130:refnum<queue>, error out=w128:errorcluster)  [unwired: 1 out]
        n28 = case shown="False" "Stop" {
          tunnel: w130 -> [w144 w149]
          tunnel: [w144 w148] -> w129
          tunnel: w128 -> [w143 w147]
          tunnel: [w143 w146] -> w127
          frame False {
          }
          frame True {
            n29 = Enqueue Element(queue=w149, element=PixieKeithleyDAQstates."Stop", error in (no error)=w147) -> (queue out=w148:refnum<queue>, error out=w146:errorcluster)  [unwired: 2 out]
          }
        }
        n30 = case shown="False" "StartDAQ" {
          tunnel: [PixieKeithleyDAQstates."Idle" ("element") PixieKeithleyDAQstates."Start Run" ("element")] -> w135
          frame False {
            n31 = Wait (ms)(milliseconds to wait=u32 10) -> ()  [unwired: 1 out]
          }
          frame True {
          }
        }
        n32 = Enqueue Element(queue=w129, element=w135, error in (no error)=w127) -> (error out=w132:errorcluster)  [unwired: 3 out]
        n33 = case shown="\"Tuning\"" "Mode" {
          frame "Tuning" {
            n34 = property on="Run Parameters" class="Clust (strict)"("Value"=T5 {"Block time (s)"=0.2, "Max Runtime (s)"=100000.0, "Max Counts"=100000, "C12 Limit"=-1.0, "Max BadBlocks"=100} ("Run Parameters")) -> ()  [unwired: 2 in, 2 out]
          }
          frame "Manual" {
          }
          frame "Run", Default {
            n35 = property on="Run Parameters" class="Clust (strict)"("Value"=T5 {"Block time (s)"=1.0, "Max Runtime (s)"=10.0, "Max Counts"=100000, "C12 Limit"=-1.0, "Max BadBlocks"=0} ("Run Parameters")) -> ()  [unwired: 2 in, 2 out]
          }
        }
      }
      frame "Start Run" {
        w163 = T4[] [enum."Wait", enum."Get Block", enum."Check Data"] items=["Initialize", "Restart Bouncer", "Idle", "Load Wheel", "Load Sample", "Start Run", "Wait", "Get Block", "Check Data", "Check Run", "Check Sample", "Analyse and Display", "Stop DAQ", "Log Data", "Stop"]
        w167 = TRUE
        # "Start Bouncer and Gate\nTrigger DAQ and PIXIE"
        # "Start counter"
        # "Code to trigger sync start goes here"
        # "Start/trigger PIXIE"
        # "Start FC DAQ"
        n36 = Not(x=w167) -> (.not. x?=w168:bool)
        n37 = shared-variable "My Computer\\NOSAMSPixieDAQVars.lvlib\\StartDAQ"(w168, error in=w154) -> (error out=w159:errorcluster)
        n38 = call "PixieStartACQ.vi"("error in (no error)"=w159) -> ("error out"=w172:errorcluster)  [unwired: 2 in, 8 out]
        n39 = call <vilib>:"DAQmx Start Task.vi"("task/channels in"=w161, "error in"=w159) -> ("task out"=w160:refnum<k21>, "error out"=w158:errorcluster)  [unwired: 12 out]
        n40 = call "ElapsedTime.vi"("error in (no error)"=w159, "Mode (Update)"=enum16{"Update", "Init"}."Init") -> ("error out"=w171:errorcluster)  [unwired: 9 out]
        n41 = Merge Errors(w171, w172, w158) -> (w166:errorcluster)
        n42 = for {
          tunnel: w169 -> [w178]
          tunnel: w166 -> [w177]
          tunnel: [w176] -> w165
          tunnel: w163 -> [w175] mode=indexing
          n43 = Enqueue Element(queue=w178, element=w175, error in (no error)=w177) -> (error out=w176:errorcluster)  [unwired: 3 out]
        }
        "Acquiring" <- w167
      }
      frame "Wait" {
        # "Wait for pixie and SRS to get one block of data"
        n44 = disable-structure shown="Disabled" {
          disable-tunnel: [w198 _] -> w184
          disable-tunnel: w183 -> [w197 _]
          disable-tunnel: w181 -> [w196 _]
          disable-tunnel: [w195 _] -> w180
          frame Disabled {
            # "Start Cups"
            n45 = call <vilib>:"DAQmx Start Task.vi"("task/channels in"=w196, "error in"=w197) -> ("task out"=w195:refnum<k21>, "error out"=w198:errorcluster)  [unwired: 12 out]
          }
          frame Enabled {
          }
        }
        n46 = Unbundle By Name(w189) -> ("Block time (s)"=w191:dbl)
        n47 = Multiply(x=w191, y=1000.0) -> (x*y=w190:dbl)
        n48 = flat-sequence {
          tunnel: w190 -> [w200]
          tunnel: w184 -> [w199]
          tunnel: [w199] -> w182
          frame #0 {
            n49 = Wait (ms)(milliseconds to wait=w200) -> ()  [unwired: 1 out]
          }
        }
      }
      frame "Get Block" {
        w221 = 10171 items=["Rising"=10280, "Falling"=10171] ("slope")
        w216 = 10178 items=["Finite Samples"=10178, "Continuous Samples"=10123] ("sample mode")
        # "LT&RT won't be accurate unless PIXIE is stopped."
        # "Problem: PIXIE & FCs not synched."
        n50 = call-poly <vilib>:"DAQmx Create Virtual Channel.vi"("maximum value"=10.0 ("minimum value"), "minimum value"=-10.0, "physical channels"=tag "PXI1Slot4/ai0:4", "error in"=w203) -> ("task out"=w215:refnum<k21>, "error out"=w214:errorcluster)  [unwired: 5 in, 5 out]
        n51 = call-poly <vilib>:"DAQmx Timing.vi"("task/channels in"=w215, "sample mode"=w216, "samples per channel"=1000, "rate"=100000.0, "error in"=w214) -> ("task out"=w217:refnum<k21>, "error out"=w218:errorcluster)  [unwired: 2 in, 7 out]
        n52 = call-poly <vilib>:"DAQmx Trigger.vi"("task/channels in"=w217, "source"=tag "/PXI1Slot4/PFI13", "edge"=w221, "error in"=w218) -> ("task out"=w205:refnum<k21>, "error out"=w204:errorcluster)  [unwired: 1 in, 9 out]
        n53 = disable-structure shown="Disabled" {
          disable-tunnel: w268 -> [w276 _]
          disable-tunnel: w203 -> [w273 _]
          disable-tunnel: [w271 _] -> w223
          disable-tunnel: [w269 _] -> _
          frame Disabled {
            # "Stop cups"
            n54 = call-poly <vilib>:"DAQmx Read.vi"("task/channels in"=w276, "number of samples per channel"=-1, "timeout"=10.0, "error in"=w273) -> ("task out"=w272:refnum<k21>, "error out"=w270:errorcluster)  [unwired: 10 out]
            n55 = call <vilib>:"DAQmx Stop Task.vi"("task/channels in"=w272, "error in"=w270) -> ("task out"=w271:refnum<k21>, "error out"=w269:errorcluster)  [unwired: 12 out]
          }
          frame Enabled {
          }
        }
        n56 = call <vilib>:"DAQmx Start Task.vi"("task/channels in"=w205, "error in"=w204) -> ("task out"=w212:refnum<k21>, "error out"=w211:errorcluster)  [unwired: 12 out]
        n57 = call-poly <vilib>:"DAQmx Read.vi"("task/channels in"=w212, "error in"=w211) -> ("task out"=w210:refnum<k21>, "data"=w201:waveform(dbl)[], "error out"=w209:errorcluster)  [unwired: 2 in, 9 out]
        "Waveform Chart" <- w201
        n58 = call "ProcessFCCurrentsLE.vi"("FC Data"=w201, "Bouncer Settings"=w222, "FC Offset"="FC Offset") -> ("Mean Currents"=w252:dbl[], "Output Waveforms"=w253:waveform(dbl)[])  [unwired: 7 in]
        n59 = Index Array(array=w253) -> (element #1=→"HE 12C Cup":waveform(dbl), element #2=→"LE 12C Cup":waveform(dbl), element #3=→"HE 13CH Cup":waveform(dbl), element #4=→"HE 13CL Cup":waveform(dbl), element #5=→"LE 13C Cup":waveform(dbl), element #6=→"Bouncer":waveform(dbl))  [unwired: 6 in]
        n60 = Index Array(array=w252) -> (element #1=w242:dbl, element #2=w231:dbl, element #3=w241:dbl, element #4=w240:dbl, element #5=w230:dbl)  [unwired: 5 in]
        "C13H" <- w241
        "C13L" <- w240
        "C12" <- w242
        "C12LE" <- w231
        "C13LE" <- w230
        n61 = call <vilib>:"DAQmx Clear Task.vi"("task in"=w210, "error in"=w209) -> ("error out"=w202:errorcluster)  [unwired: 13 in]
        n62 = Add(x=w241, y=w240) -> (x+y=w250:dbl)
        n63 = Divide(x=w241, y=w240) -> (x/y=→"13C H/L":dbl)
        n64 = call "PixieGetData.vi"("error IO"=w202) -> ("error out"=w246:errorcluster, "PixieTimes"=w254:T9, "Histogram Data"=w235:u32[][], 3:w260, 4:w236, 5:w263, 6:→"CH0 SFDT", 7:w237, 11:→"CH0 GDT")  [unwired: 2 in]
        "Block Spectrum" <- w263
        "Ch0 LT" <- w260
        "Ch1 LT" <- w235
        "Run time [s]" <- w254
        "CH1 SFDT" <- w236
        "CH1 GDT" <- w237
        n65 = Bundle(w242, w250) -> (→"Currents":cluster{dbl, dbl})  [unwired: 1 out]
        n66 = property on="Block Spectrum" class="WFGraph (strict)"() -> ("CrsrList"=w262:T10)  [unwired: 2 in, 2 out]
        n67 = call "PixieCalcCountData.vi"("CrsrList"=w262, "Histogram Data"=w263, "CH0 LT"=w260, "CH1 LT"=w235) -> ("Count Data"=w261:T11)  [unwired: 1 in]
        n68 = Unbundle By Name(w261) -> ("Ch0 Counts"=→"Ch0 Counts":u32, "Ch0 Rate"=→"Ch0 Rate":dbl, "Ch1 Counts"=w234:u32, "Ch1 Rate"=→"Ch1 Rate":dbl)
        "Ch1 Counts" <- w234
        n69 = Add(x=w236, y=w237) -> (x+y=w238:dbl)
        n70 = Subtract(x=w235, y=w238) -> (x-y=w233:dbl[][])
        n71 = call "InsertBlockData.vi"("C12LE"=w231, "C12"=w242, "Block Data In"=w247, "C13H"=w241, "C13L"=w240, "C13LE"=w230, "Counts"=w234, "LT"=w233, "RT"=w254) -> ("Block Data Out"=w264:T8)  [unwired: 6 in]
        n72 = Divide(x=w234, y=w233) -> (x/y=w232:dbl[][])
        "DT Corrected Rate" <- w232
        n73 = Bundle(w242, w250, w232, w231, w230) -> (→"Currents & Counts":cluster{dbl, dbl, dbl[][], dbl, dbl})  [unwired: 1 out]
      }
      frame "Check Data" {
        # "check if stats reqs satisfied\nwrite to logfile"
        # "Check block data"
        # "Check data quality\n    add to run data if good\n    discard, increment bad block counter\n     get new block if bad"
        n74 = Unbundle By Name(w289) -> ("C12"=w292:dbl[])
        n75 = Unbundle By Name(w285) -> ("C12 Limit"=w294:dbl, "Max BadBlocks"=w288:u8)
        n76 = case shown="False" "Stop DAQ" {
          tunnel: w287 -> [w296 w299]
          tunnel: [w296 w298] -> w286
          frame False {
          }
          frame True {
            n77 = Enqueue Element(queue=w299, element=PixieKeithleyDAQstates."Stop DAQ" ("Next State")) -> (queue out=w298:refnum<queue>)  [unwired: 1 in, 3 out]
          }
        }
        n78 = Delete From Array(array=w292) -> (deleted portion=w291:dbl)  [unwired: 2 in, 1 out]
        n79 = Greater?(x=w291, y=w294) -> (0:w290:bool)
        "Good Block" <- w290
        n80 = case shown="True" w290 {
          tunnel: [w309 w313] -> w279
          tunnel: w278 -> [w310 w314]
          tunnel: w289 -> [_ w315]
          tunnel: w288 -> [w308 _]
          tunnel: w286 -> [w306 w317]
          frame False {
            w303 = T4[] [enum."Wait", enum."Get Block", enum."Check Data"] items=["Initialize", "Restart Bouncer", "Idle", "Load Wheel", "Load Sample", "Start Run", "Wait", "Get Block", "Check Data", "Check Run", "Check Sample", "Analyse and Display", "Stop DAQ", "Log Data", "Stop"]
            w305 = T4[] [enum."Stop DAQ"] items=["Initialize", "Restart Bouncer", "Idle", "Load Wheel", "Load Sample", "Start Run", "Wait", "Get Block", "Check Data", "Check Run", "Check Sample", "Analyse and Display", "Stop DAQ", "Log Data", "Stop"]
            # "Bad Block"
            n81 = Unbundle By Name(w310) -> ("BadBlocks"=w302:u8)
            n82 = Decrement(x=w308) -> (x-1=w301:u8)
            n83 = Increment(x=w302) -> (x+1=w300:u8)
            n84 = Bundle By Name(cluster=w310, "BadBlocks"=w300) -> (w309:T3)
            n85 = Greater Or Equal?(x=w300, y=w301) -> (x >= y?=w307:bool)
            n86 = Select(t=w305, s=w307, f=w303) -> (s? t:f=w304:T4[])
            n87 = for {
              tunnel: w304 -> [w312] mode=indexing
              tunnel: w306 -> [w311]
              n88 = Enqueue Element(queue=w311, element=w312) -> ()  [unwired: 1 in, 4 out]
            }
          }
          frame True {
            n89 = call "PKDAQAppendBlockDataCont.vi"("Run Summary"=w314, "Block Data"=w315) -> ("Run Summary Out"=w313:T3)  [unwired: 9 out]
            n90 = Enqueue Element(queue=w317, element=PixieKeithleyDAQstates."Check Run") -> ()  [unwired: 1 in, 4 out]
          }
        }
        "Summary Data" <- w279
      }
      frame "Check Run" {
        # "Get another block?"
        n91 = Unbundle By Name(w325) -> ("Max Counts"=w335:u32, "Max Runtime (s)"=w334:dbl)
        n92 = Unbundle By Name(w329) -> ("Counts"=w331:u32, "LT"=w330:dbl)
        n93 = Less?(x=w335, y=w331) -> (x < y?=w327:bool)
        n94 = Greater Or Equal?(x=w330, y=w334) -> (x >= y?=w326:bool)
        n95 = Or(x=w327, y=w326) -> (x .or. y?=w328:bool)
        n96 = case shown="True" w328 {
          tunnel: [w339 w340] -> w324
          frame False {
            w339 = T4[] [enum."Analyse and Display", enum."Wait", enum."Get Block", enum."Check Data"] items=["Initialize", "Restart Bouncer", "Idle", "Load Wheel", "Load Sample", "Start Run", "Wait", "Get Block", "Check Data", "Check Run", "Check Sample", "Analyse and Display", "Stop DAQ", "Log Data", "Stop"]
          }
          frame True {
            w340 = T4[] [enum."Analyse and Display", enum."Stop DAQ"] items=["Initialize", "Restart Bouncer", "Idle", "Load Wheel", "Load Sample", "Start Run", "Wait", "Get Block", "Check Data", "Check Run", "Check Sample", "Analyse and Display", "Stop DAQ", "Log Data", "Stop"]
          }
        }
        n97 = for {
          tunnel: w323 -> [w338]
          tunnel: w324 -> [w337] mode=indexing
          n98 = Enqueue Element(queue=w338, element=w337) -> ()  [unwired: 1 in, 4 out]
        }
      }
      frame "Analyse and Display" {
        n99 = call "PKDAQRunningAvg.vi"("Block Data"=w342, "CountPoints"="CountPoints", "CurPoints"="CurPoints") -> ("RunningAverages"=w360:T3)  [unwired: 8 out]
        "RunningAverages" <- w360
        n100 = call "CalcRatiosBouncer.vi"("Run Summary"=w360) -> ("Run Ratios"=w356:T7)  [unwired: 10 out]
        "Moving Averages" <- w356
        n101 = call "CalcRatiosBouncer.vi"("Run Summary"=w343) -> ("Run Ratios"=w347:T7)  [unwired: 10 out]
        "Run Average Ratios" <- w347
        n102 = Unbundle By Name(w347) -> ("C14Rate"=w359:dbl)
        n103 = Unbundle By Name(w356) -> ("C14Rate"=w357:dbl)
        n104 = Unbundle By Name(w347) -> ("C14/12"=w355:dbl, "d13C"=w350:dbl)
        n105 = Unbundle By Name(w356) -> ("C14/12"=w354:dbl, "d13C"=w349:dbl, "C13/12"=w353:dbl)
        n106 = Reciprocal(x=w353) -> (1/x=→"12/13":dbl)
        n107 = Bundle("C14Rate"=w359, "C14Rate"=w357) -> (→"Ch1 Rate 2":cluster{"C14Rate":dbl, "C14Rate":dbl})  [unwired: 1 out]
        n108 = Bundle("C14/12"=w355, "C14/12"=w354, "d13C"=w350, "d13C"=w349) -> (→"Ratios":T6)  [unwired: 1 out]
      }
      frame "Stop DAQ" {
        n109 = call "PixieStopACQ.vi"("error in (no error)"=w372) -> ("error out"=w376:errorcluster)  [unwired: 10 out]
        n110 = call "PixieCheckRunStatus.vi"("error in (no error)"=w376) -> ("error out"=w370:errorcluster, "run finished"=w375:bool)  [unwired: 1 in, 8 out]
        n111 = case shown="True" w375 {
          tunnel: w374 -> [w380 w382]
          frame False {
            n112 = Enqueue Element(queue=w380, element=PixieKeithleyDAQstates."Stop DAQ" ("Next State")) -> ()  [unwired: 1 in, 4 out]
          }
          frame True {
            w381 = T4[] [enum."Get Block", enum."Check Data", enum."Analyse and Display", enum."Log Data", enum."Idle"] items=["Initialize", "Restart Bouncer", "Idle", "Load Wheel", "Load Sample", "Start Run", "Wait", "Get Block", "Check Data", "Check Run", "Check Sample", "Analyse and Display", "Stop DAQ", "Log Data", "Stop"]
            n113 = for {
              tunnel: w382 -> [w384]
              tunnel: w381 -> [w383] mode=indexing
              n114 = Enqueue Element(queue=w384, element=w383) -> ()  [unwired: 1 in, 4 out]
            }
          }
        }
      }
      frame "Log Data" {
        # "Add data to status file and return here?"
        # "Return to DAQ Control\nData if good run\nError condition if bad"
        n115 = call "ElapsedTime.vi"("error in (no error)"=w396) -> ("error out"=w395:errorcluster, "Elapsed Time"=w394:dbl)  [unwired: 1 in, 8 out]
        "Elapsed Time" <- w394
        n116 = call-poly <vilib>:"DAQmx Read.vi"("task/channels in"=w400, "error in"=w395) -> ("task out"=w399:refnum<k21>, "data"=w393:u32, "error out"=w398:errorcluster)  [unwired: 1 in, 10 out]
        "SCA Counts" <- w393
        n117 = call <vilib>:"DAQmx Stop Task.vi"("task/channels in"=w399, "error in"=w398) -> ("task out"=w397:refnum<k21>, "error out"=w389:errorcluster)  [unwired: 12 out]
        n118 = Unbundle By Name(w406) -> ("d13C"=w405:dbl, "C14/12"=w404:dbl)
        n119 = Unbundle By Name(w391) -> ("C12"=w419:dbl, "C13L"=w403:dbl, "C13H"=w401:dbl, "Counts"=w418:u32, "LT"=w417:dbl, "RT"=w416:dbl)
        n120 = shared-variable "My Computer\\NOSAMSPixieDAQVars.lvlib\\C13HCur"(w401) -> ()  [unwired: 2 out]
        n121 = shared-variable "My Computer\\NOSAMSPixieDAQVars.lvlib\\C12Cur"(w419) -> ()  [unwired: 2 out]
        n122 = shared-variable "My Computer\\NOSAMSPixieDAQVars.lvlib\\C13LCur"(w403) -> ()  [unwired: 2 out]
        n123 = shared-variable "My Computer\\NOSAMSPixieDAQVars.lvlib\\Runtime"(w416) -> ()  [unwired: 2 out]
        n124 = shared-variable "My Computer\\NOSAMSPixieDAQVars.lvlib\\Livetime"(w417) -> ()  [unwired: 2 out]
        n125 = shared-variable "My Computer\\NOSAMSPixieDAQVars.lvlib\\Counts"(w418) -> ()  [unwired: 2 out]
        n126 = shared-variable "My Computer\\NOSAMSPixieDAQVars.lvlib\\d13C"(w405) -> ()  [unwired: 1 in, 1 out]
        n127 = shared-variable "My Computer\\NOSAMSPixieDAQVars.lvlib\\C1412"(w404) -> ()  [unwired: 1 in, 1 out]
        n128 = Add(x=w403, y=w401) -> (x+y=w402:dbl)
        n129 = Divide(x=w393, y=w394) -> (x/y=→"SCA Rate":dbl)
        n130 = shared-variable "My Computer\\NOSAMSPixieDAQVars.lvlib\\C13"(w402) -> ()  [unwired: 1 in, 1 out]
        n131 = Build Path(base path="Log File Path", name or relative path="Logfile") -> (appended path=w410:path)
        n132 = call "CreateLogfile.vi"("error in (no error)"=w389, "Log File Path"=w410) -> ("error out"=w420:errorcluster)  [unwired: 1 in, 8 out]
        n133 = call "BouncerDAQinit.vi"("error in (no error)"=w420) -> ("error out"=w387:errorcluster, "Run Ratios"=w409:T7, "Summary Data"=w408:T3, "Block Data"=w407:T8)  [unwired: 1 in, 6 out]
        n134 = shared-variable "My Computer\\NOSAMSPixieDAQVars.lvlib\\Acquiring"(FALSE ("Acquire"), error in=w387) -> (error out=w413:errorcluster)
      }
      frame "Stop" {
        n135 = Enqueue Element(queue=w429, element=PixieKeithleyDAQstates."Stop" ("Next State")) -> ()  [unwired: 1 in, 4 out]
      }
    }
    n136 = Equal?(x=w37, y=PixieKeithleyDAQstates."Stop" ("States")) -> (x = y?=w52:bool)
  }
  n137 = call <vilib>:"DAQmx Clear Task.vi"("task in"=w4, "error in"=w2) -> ("error out"=w3:errorcluster)  [unwired: 13 out]
  n138 = call <vilib>:"DAQmx Clear Task.vi"("task in"=w5, "error in"=w3) -> ("error out"=w1:errorcluster)  [unwired: 13 out]
  n139 = call <vilib>:"DAQmx Clear Task.vi"("task in"=w26, "error in"=w1) -> ("error out"=w8:errorcluster)  [unwired: 13 out]
  n140 = call <vilib>:"DAQmx Clear Task.vi"("task in"=w6, "error in"=w8) -> ("error out"=w7:errorcluster)  [unwired: 13 out]
  n141 = Release Queue(queue=w20, error in (no error)=w7) -> (error out=w13:errorcluster)  [unwired: 3 out]
  n142 = call <vilib>:"General Error Handler.vi"("error in (no error)"=w13) -> ("error out"=→"error out":errorcluster)  [unwired: 1 in, 13 out]
